vi "Write Cycle - Single DUT.vi"(0 "Cycle Instructions":T1[](array[typedef]) {"Post CMD Delay (s)" format="%#_4ps"; "DAC Vout (V)" format="%.3f V"; "Dev Ch Idx (0-5)" max=5 step=1 format="Ch %d"}, 11 "error in":errorcluster, 12 "Log (T)":bool=TRUE, 13 "DUT":T3, 14 "FPGA":T2) -> (15 "error out":errorcluster)   [LabVIEW 2017, in "Host SRL.lvlib"]
uses:
  Host SRL.lvlib
  Type Defs/WSVCAP SHL DUT Number Enum.ctl
  Type Defs/WSVCAP SHL FPGA Enum.ctl
  Type Defs/Cycle Instruction Cluster.ctl
panel:
  out "Socket Mask":u32=1 format="%06x"
  out "SRL Data Out":u8[][](array[numeric]) format="%02x"
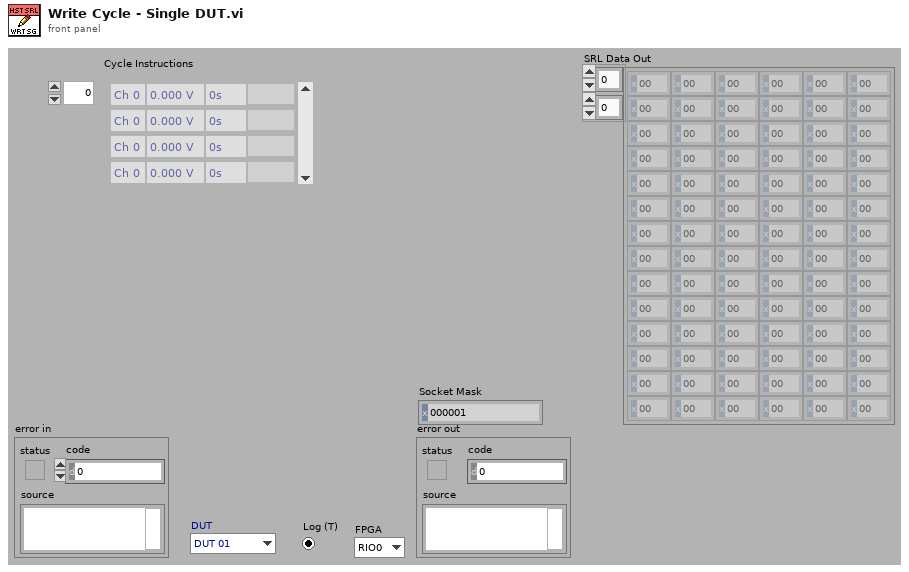
[diagram p1: front panel]
types:
  T1 = typedef "Host SRL.lvlib/Cycle Instruction Cluster.ctl" = cluster{"Dev Ch Idx (0-5)":u32, "DAC Vout (V)":dbl, "Post CMD Delay (s)":dbl, "Raw CMD":string}
  T2 = typedef "WSVCAP SHL FPGA Enum.ctl" = enum16{"RIO0", "RIO1"}
  T3 = typedef "WSVCAP SHL DUT Number Enum.ctl" = enum16{"DUT 01", "DUT 02", "DUT 03", "DUT 04", "DUT 05", "DUT 06", "DUT 07", "DUT 08", "DUT 09", "DUT 10", "DUT 11", "DUT 12", "DUT 13", "DUT 14", "DUT 15", "DUT 16", "DUT 17", "DUT 18", "DUT 19", "DUT 20", "DUT 21", "DUT 22", "DUT 23", "DUT 24"}
  T4 = typedef "WSVCAP SHL Core System Cluster.ctl" = cluster{"Settings":T5, "FPGA Resource":tag, "Online":bool, "I2C Wait Ticks":u32, "SRL Wait Ticks":u32, "FPGA VI Reference (FPGA Mode)":T6, "FPGA VI Reference (Sim Mode)":refnum<vi>}
  T5 = typedef "WSVCAP SHL I2C Settings Cluster.ctl" = cluster{"I2C Slave Address":u8, "I2C Clock Rate (Hz)":dbl, "SRL Clock Rate (Hz)":dbl, "Simulate FPGA":bool, "C1 Cap DAC Default":u8, "C2 Cap DAC Default":u8, "C3 Cap DAC Default":u8, "C4 Cap DAC Default":u8, "DAC Out Vref (V)":dbl}
  T6 = typedef "WSVCAP SHL FPGA Ref.ctl" = refnum<k20>
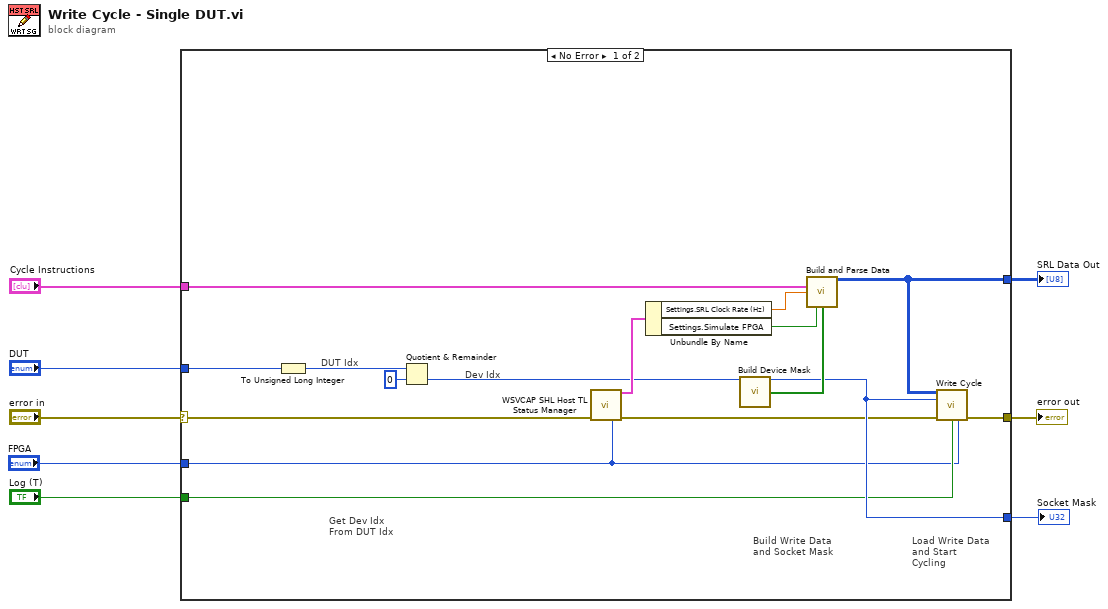
[diagram p0: block diagram]
diagram:
  n1 = case shown="No Error" "error in" {
    selector: "error in" -> [w13 _]
    tunnel: [w22 _] -> w8
    tunnel: [w16 _] -> w6
    tunnel: "DUT" -> [w12 _]
    tunnel: [w23 _] -> w4
    tunnel: "Log (T)" -> [w17 _]
    tunnel: "FPGA" -> [w15 _]
    tunnel: "Cycle Instructions" -> [w14 _]
    frame No Error {
      # "DUT Idx"
      # "Dev Idx"
      # "Get Dev Idx\nFrom DUT Idx"
      # "Load Write Data and Start Cycling"
      # "Build Write Data and Socket Mask"
      n2 = To Unsigned Long Integer(number=w12) -> (unsigned 32bit integer=w10:u32)
      n3 = Quotient & Remainder(x=w10, y=u32 0 ("Device Idx (0-5)")) -> (floor(x/y)=w9:u32)  [unwired: 1 out]
      n4 = call "WSVCAP SHL Host TL Status Manager.vi"("error in"=w13, "FPGA"=w15) -> ("System Out"=w20:T4, "error out"=w21:errorcluster)  [unwired: 12 in]
      n5 = Unbundle By Name(w20) -> ("Settings.SRL Clock Rate (Hz)"=w18:dbl, "Settings.Simulate FPGA"=w19:bool)
      n6 = call "Build Device Mask.vi"("Device Idx (0-5)"=w9) -> ("Socket Mask [U32]"=w23:u32, "DUT Mask"=w24:bool[])  [unwired: 13 in]
      n7 = call "Build and Parse Data.vi"("Cycle Instructions"=w14, "Clock Rate (Hz) (Cycle Only)"=w18, "Simulate FPGA (Cycle Only)"=w19, "Dev Mask (All)"=w24) -> ("SRL Data Out [U8]"=w16:u8[][])  [unwired: 10 in, 1 out]
      n8 = call "Write Cycle.vi"("SRL Data Out"=w16, "Socket Mask"=w23, "error in"=w21, "Log (T)"=w17, "FPGA"=w15) -> ("error out"=w22:errorcluster)  [unwired: 10 in]
    }
    frame Error {
    }
  }
  "error out" <- w8
  "SRL Data Out" <- w6
  "Socket Mask" <- w4
